vi "Grab.vi"() -> ()   [LabVIEW 2011]
doc: "The Grab VI acquires images continuously and displays the images in an image control using high-level acquisition VIs. A grab is appropriate for high-speed applications in which you need to process only one image at a time."
uses:
  <vilib>/vision/driver/NI_Vision_Acquisition_Software.lvlib
panel:
  in  "Camera Name":refnum<k21> caption="IMAQdx Session"
  out "Buffer Number":u32
  out "Image":T1(plugin-control)
  out "Frame Rate":dbl(knob) scale=0.0..100.0
  in  "Stop":bool
  # "Overview: Demonstrates how to acquire images continuously using a Grab acquisition.\nRequirements: Vision Acquisition Software\nInstructions: \n1. Select the Camera Name.\n2. Run the VI"
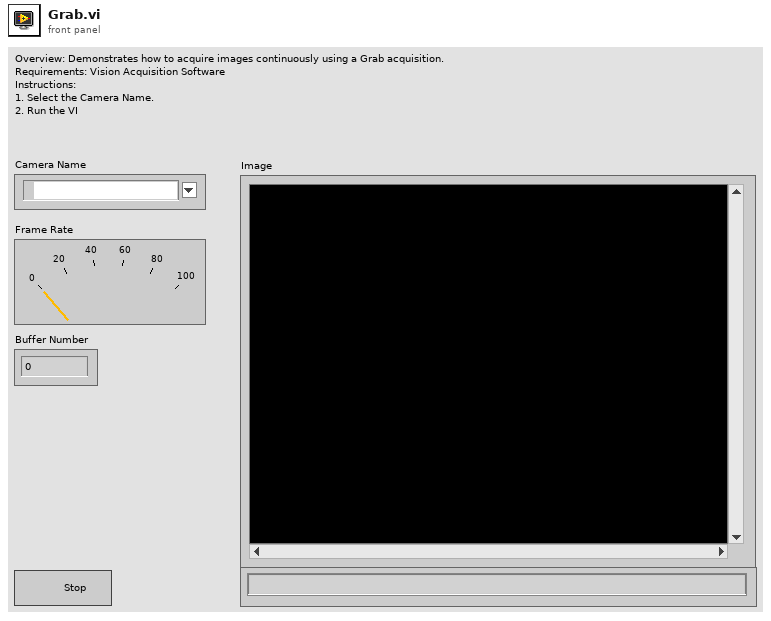
[diagram p1: front panel]
types:
  T1 = typedef "IMAQ Image.ctl" = refnum<image>
  T2 = typedef "IMAQdx.ctl" = refnum<k21>
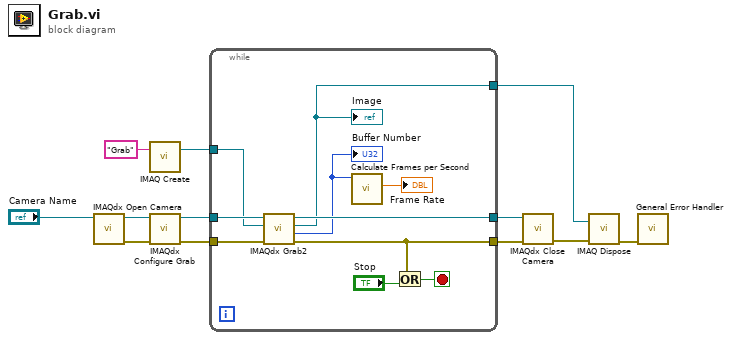
[diagram p0: block diagram]
diagram:
  n1 = call <vilib>:"IMAQdx Open Camera.vi"("Session In"="Camera Name") -> ("error out"=w7:errorcluster, "Session Out"=w6:T2)  [unwired: 2 in, 7 out]
  n2 = call "IMAQ Create"("Image Name"="Grab") -> ("New Image"=w12:T1)  [unwired: 3 in, 2 out]
  n3 = call <vilib>:"IMAQdx Configure Grab.vi"("error in"=w7, "Session In"=w6) -> ("error out"=w10:errorcluster, "Session Out"=w11:T2)  [unwired: 8 out]
  n4 = while {
    tunnel: [w17] -> w9
    tunnel: w10 -> [w19]
    tunnel: w11 -> [w20]
    tunnel: [w14] -> w8
    tunnel: w12 -> [w18]
    tunnel: [w13] -> w4
    stop <- w22 stop-if-true
    n5 = call <vilib>:"IMAQdx Grab2.vi"("error in"=w19, "Image In"=w18, "Session In"=w20) -> ("error out"=w14:errorcluster, "Buffer Number Out"=w15:u32, "Image Out"=w13:T1, "Session Out"=w17:T2)  [unwired: 5 in]
    "Image" <- w13
    "Buffer Number" <- w15
    n6 = call <vilib>:"Calculate Frames per Second.vi"("Buffer Number"=w15) -> ("Processed Frames/s"=→"Frame Rate":dbl)  [unwired: 8 in, 2 out]
    n7 = Or(x=w14, y="Stop") -> (x .or. y?=w22:bool)
  }
  n8 = call <vilib>:"IMAQdx Close Camera.vi"("error in"=w8, "Session In"=w9) -> ("error out"=w3:errorcluster)  [unwired: 9 out]
  n9 = call "IMAQ Dispose"("Image"=w4, "error in (no error)"=w3) -> ("error out"=w2:errorcluster)  [unwired: 4 in]
  n10 = call <vilib>:"General Error Handler.vi"("error in (no error)"=w2) -> ()  [unwired: 1 in, 14 out]
